vi "TCP_send.vi"(8 "error in (no error)":errorcluster) -> (0 "error out":errorcluster)   [LabVIEW 2013, in "TCP_IP.lvclass"]
uses:
  TCP_IP.lvclass
  Globals.vi
panel:
  out "Return Data":string
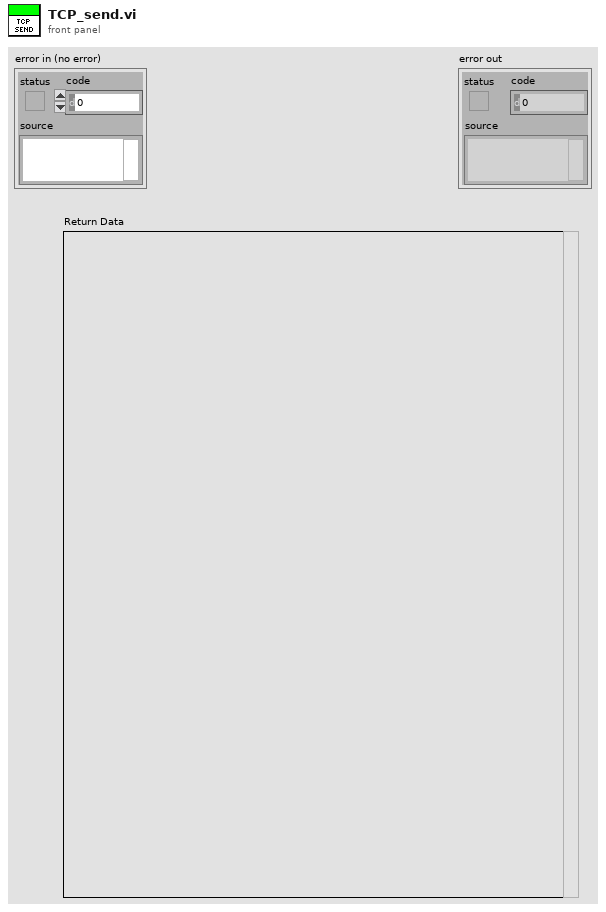
[diagram p1: front panel]
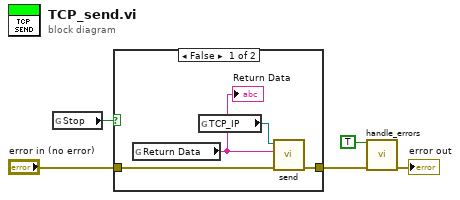
[diagram p0: block diagram]
diagram:
  n1 = global read "Globals.vi" "Stop"() -> (w2:bool)
  n2 = case shown="False" w2 {
    tunnel: [w9 w10] -> w5
    tunnel: "error in (no error)" -> [w7 w10]
    frame False {
      n3 = global read "Globals.vi" "Return Data"() -> (w6:string)
      "Return Data" <- w6
      n4 = global read "Globals.vi" "TCP_IP"() -> (w8:refnum<class "TCP_IP.lvclass">)
      n5 = call "send.vi"("error in (no error)"=w7, "messge"=w6, "TCP_IP (in)"=w8) -> ("error out"=w9:errorcluster)  [unwired: 8 in]
    }
    frame True {
    }
  }
  n6 = call "handle_errors.vi"("Exit Operation"=TRUE ("Exit Measurement"), "error in (no error)"=w5) -> ("error out"=→"error out":errorcluster)  [unwired: 13 in]
